vi "Read Count.vi"(8 "错误输入（无错误）":errorcluster, 11 "OSC Input":refnum<visa-resource-name>) -> (0 "错误输出":errorcluster, 2 "Pace Interval":dbl, 3 "OSC Output":refnum<visa-resource-name>)   [LabVIEW 2016]
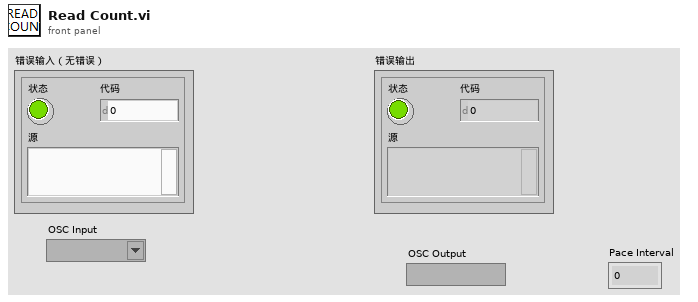
[diagram p1: front panel]
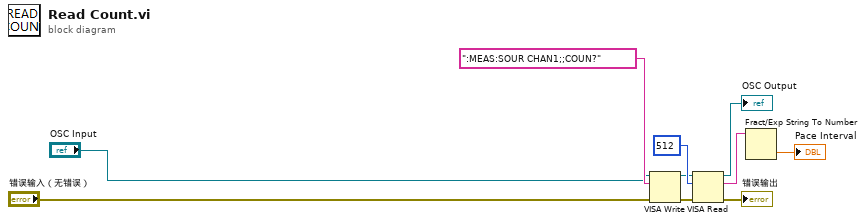
[diagram p0: block diagram]
diagram:
  n1 = VISA Write(VISA resource name="OSC Input", write buffer=":MEAS:SOUR CHAN1;;COUN?" ("写入缓冲区"), error in (no error)="错误输入（无错误）") -> (VISA resource name out=w7:refnum<visa-resource-name>, error out=w6:errorcluster)  [unwired: 1 out]
  n2 = VISA Read(VISA resource name=w7, byte count=u32 512 ("字节总数"), error in (no error)=w6) -> (VISA resource name out=→"OSC Output":refnum<visa-resource-name>, read buffer=w5:string, error out=→"错误输出":errorcluster)  [unwired: 1 out]
  n3 = Fract/Exp String To Number(string=w5) -> (number=→"Pace Interval":dbl)  [unwired: 3 in, 1 out]
